vi "Get - Vector - Reals.vi"(5 "use temporary file?":bool, 7 "data type of variable":dbl[](array[numeric]), 8 "error in":errorcluster, 10 "variable name":string, 11 "pipe in":T1) -> (0 "error out":errorcluster, 2 "value":dbl[](array[numeric]) format="%.2f", 3 "pipe out":T1)   [LabVIEW 2013, in "GOLPI library.lvlib"]
uses:
  GOLPI library.lvlib
  LV Process.lvlibp/Pipe Handle.ctl
  Custom Error Codes Enum Type Def.vi
  LV Process.lvlibp
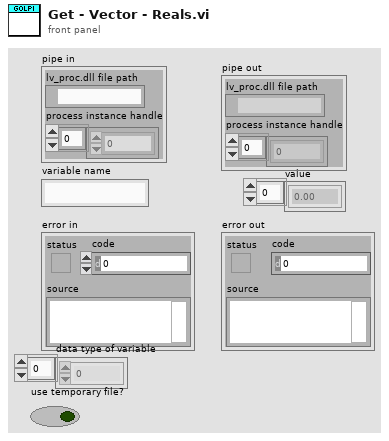
[diagram p1: front panel]
types:
  T1 = typedef "LV Process.lvlibp/Pipe Handle.ctl" = cluster{"lv_proc.dll file path":path, "process instance handle":u32[]}
  T2 = typedef "GOLPI library.lvlib/Custom Error Codes Enum Type Def.vi" = enum16{"no error", "00 working directory PAR1 missing", "01 octave binary PAR1 missing", "02 octave report error PAR1", "03 empty output last cmd PAR1", "04 missing temporary file PAR1", "10 var PAR1 not string", "11 var PAR1 not num, scal, ~compl", "12 var PAR1 not num, scal, compl", "13 var PAR1 not num, vect, ~compl", "14 var PAR1 not num, vect, compl", "15 var PAR1 not num, mat, ~compl", "16 var PAR1 not num, mat, ~compl", "99 not finished"}
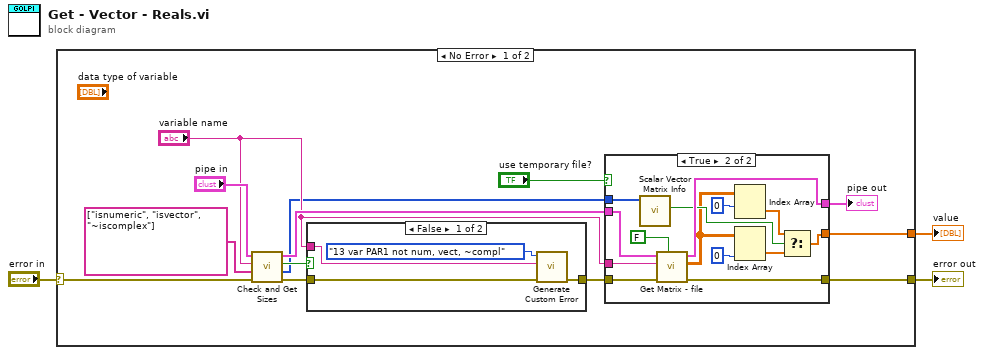
[diagram p0: block diagram]
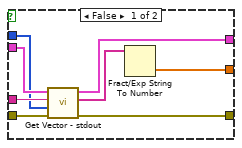
[diagram p2: hidden frame]
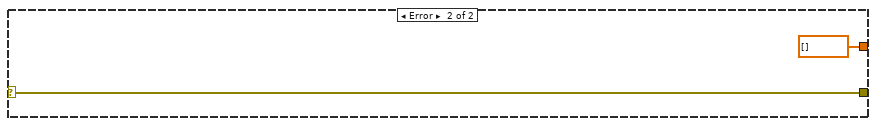
[diagram p4: hidden frame]
diagram:
  n1 = case shown="No Error" "error in" {
    selector: "error in" -> [w13 w45]
    tunnel: [w7 w45] -> w3
    tunnel: [w16 dbl[] [] ("value")] -> w1
    frame No Error {
      n2 = call "Check and Get Sizes.vi"("error in (no error)"=w13, "test commands"=string[] ["isnumeric", "isvector", "~iscomplex"], "variable name"="variable name", "pipe in"="pipe in") -> ("error out"=w12:errorcluster, "octave sizes"=w4:i32[], "all tests OK?"=w14:bool, "pipe out"=w10:T1)  [unwired: 4 in]
      n3 = case shown="False" w14 {
        tunnel: w12 -> [w41 w43]
        tunnel: [w40 w43] -> w8
        tunnel: "variable name" -> [w39 _]
        frame False {
          n4 = call "Generate Custom Error.vi"("error in"=w41, "PAR1"=w39, "Enum"=Custom_Error_Codes_Enum_Type_Def.vi."13 var PAR1 not num, vect, ~compl") -> ("error out"=w40:errorcluster)  [unwired: 8 in]
        }
        frame True {
        }
      }
      n5 = case shown="True" "use temporary file?" {
        tunnel: [w18 w29] -> w16
        tunnel: w10 -> [w24 w37]
        tunnel: [w23 w36] -> w9
        tunnel: w8 -> [w22 w34]
        tunnel: [w21 w33] -> w7
        tunnel: "variable name" -> [w19 w35]
        tunnel: w4 -> [w17 w32]
        frame False {
          n6 = call "Get Vector - stdout.vi"("error in (no error)"=w22, "octave vector sizes"=w17, "variable name"=w19, "pipe in"=w24) -> ("error out"=w21:errorcluster, "vector"=w20:string[], "pipe out"=w23:T1)  [unwired: 4 in, 1 out]
          n7 = Fract/Exp String To Number(string=w20) -> (number=w18:dbl[])  [unwired: 3 in, 1 out]
        }
        frame True {
          n8 = call "Scalar Vector Matrix Info.vi"("octave sizes"=w32) -> ("is vector?"=w31:bool)  [unwired: 5 in, 5 out]
          n9 = call "Get Matrix - file.vi"("is string"=FALSE, "error in (no error)"=w34, "variable name"=w35, "pipe in"=w37) -> ("error out"=w33:errorcluster, "double array"=w27:dbl[][], "pipe out"=w36:T1)  [unwired: 3 in, 2 out]
          n10 = Index Array(array=w27, index (row)=0) -> (element=w28:dbl[])  [unwired: 1 in]
          n11 = Index Array(array=w27, index (col)=0 ("disabled index (col)")) -> (element=w30:dbl[])  [unwired: 1 in]
          n12 = Select(t=w28, s=w31, f=w30) -> (s? t:f=w29:dbl[])
        }
      }
      "pipe out" <- w9
    }
    frame Error {
    }
  }
  "value" <- w1
  "error out" <- w3
